vi "Cluster Typedef JSON Staging.vi"() -> ()   [LabVIEW 2016]
uses:
  <userlib>/LevyLab/Lockin-Multichannel/Typedefs/AO-cluster.ctl
  <userlib>/LevyLab/Lockin-Multichannel/Typedefs/AO_Amp-array.ctl
  <userlib>/LevyLab/Lockin-Multichannel/Typedefs/AO_DC-array.ctl
  <userlib>/LevyLab/Lockin-Multichannel/Typedefs/AO_f-array.ctl
  <userlib>/LevyLab/Lockin-Multichannel/Typedefs/AO_phi-array.ctl
  <userlib>/LevyLab/Lockin-Multichannel/Typedefs/Function-array.ctl
  <userlib>/LevyLab/Lockin-Multichannel/Typedefs/Function-enum.ctl
  <userlib>/LevyLab/Krohn Hite 7008/typedefs/KH_control_array.ctl
  <userlib>/LevyLab/Krohn Hite 7008/typedefs/KH_control.ctl
  <userlib>/LevyLab/Krohn Hite 7008/typedefs/Channel-Enum.ctl
  <userlib>/LevyLab/Krohn Hite 7008/typedefs/Gain-Enum.ctl
  <userlib>/LevyLab/Krohn Hite 7008/typedefs/Shunt-Enum.ctl
  <userlib>/LevyLab/Krohn Hite 7008/typedefs/Input Configuration-Enum.ctl
  <userlib>/LevyLab/Lockin-Multichannel/Typedefs/REF-cluster.ctl
  <userlib>/LevyLab/Lockin-Multichannel/Typedefs/REF_f-array.ctl
  <userlib>/LevyLab/Lockin-Multichannel/Typedefs/REF_phi-array.ctl
  <vilib>/addons/_JKI.lib/Serialization/JSON/JKI JSON Serialization.lvlib
  <userlib>/LevyLab/Krohn Hite 7008/KH7008.lvclass
panel:
  out "x = y?":T1
  out "from JSON (ms)":u32
  out "to JSON (ms)":u32
  out "JSON String":string
  in  "Experiment Description":T2
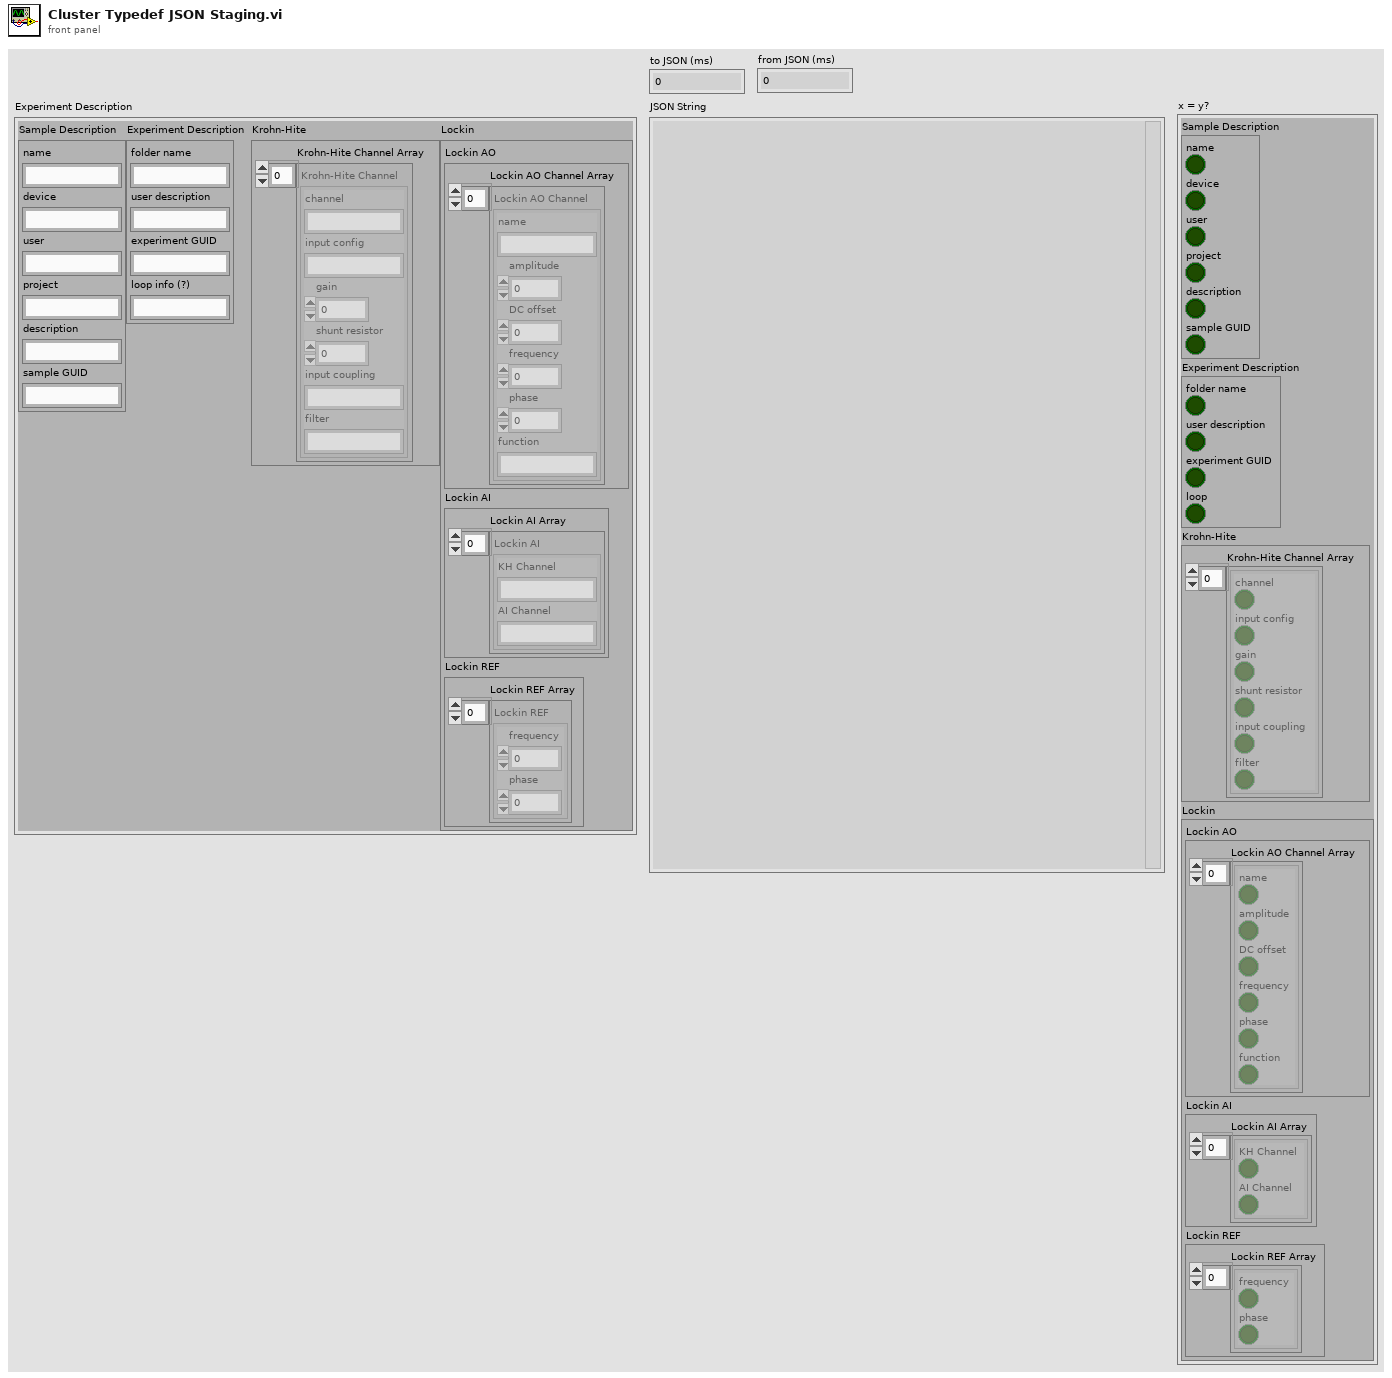
[diagram p1: front panel]
types:
  T1 = cluster{"Sample Description":cluster{"name":bool, "device":bool, "user":bool, "project":bool, "description":bool, "sample GUID":bool}, "Experiment Description":cluster{"folder name":bool, "user description":bool, "experiment GUID":bool, "loop":bool}, "Krohn-Hite":cluster{"Krohn-Hite Channel Array":cluster{"channel":bool, "input config":bool, "gain":bool, "shunt resistor":bool, "input coupling":bool, "filter":bool}[]}, "Lockin":cluster{"Lockin AO":cluster{"Lockin AO Channel Array":cluster{"name":bool, "amplitude":bool, "DC offset":bool, "frequency":bool, "phase":bool, "function":bool}[]}, "Lockin AI":cluster{"Lockin AI Array":cluster{"KH Channel":bool, "AI Channel":bool}[]}, "Lockin REF":cluster{"Lockin REF Array":cluster{"frequency":bool, "phase":bool}[]}}}
  T2 = cluster{"Sample Description":cluster{"name":string, "device":string, "user":string, "project":string, "description":string, "sample GUID":string}, "Experiment Description":cluster{"folder name":string, "user description":string, "experiment GUID":string, "loop info (?)":string}, "Krohn-Hite":cluster{"Krohn-Hite Channel Array":cluster{"channel":string, "input config":string, "gain":i32, "shunt resistor":i32, "input coupling":string, "filter":string}[]}, "Lockin":cluster{"Lockin AO":cluster{"Lockin AO Channel Array":cluster{"name":string, "amplitude":dbl, "DC offset":dbl, "frequency":dbl, "phase":dbl, "function":string}[]}, "Lockin AI":cluster{"Lockin AI Array":cluster{"KH Channel":string, "AI Channel":string}[]}, "Lockin REF":cluster{"Lockin REF Array":cluster{"frequency":dbl, "phase":dbl}[]}}}
  T3 = typedef "REF-cluster.ctl" = cluster{"REF f (Hz)":T4, "REF phi (°)":T5}
  T4 = typedef "REF_f-array.ctl" = dbl[]
  T5 = typedef "REF_phi-array.ctl" = dbl[]
  T6 = typedef "KH7008.lvclass/KH_control_array.ctl" = T7[]
  T7 = typedef "KH7008.lvclass/KH_control.ctl" = cluster{"Channel":T8, "Gain":T9, "Shunt Resistor":T10, "Input Config":T11}
  T8 = typedef "KH7008.lvclass/Channel-Enum.ctl" = enum16{"Channel 1", "Channel 2", "Channel 3", "Channel 4", "Channel 5", "Channel 6", "Channel 7", "Channel 8"}
  T9 = typedef "KH7008.lvclass/Gain-Enum.ctl" = enum16{"1x", "10x", "100x", "1000x"}
  T10 = typedef "KH7008.lvclass/Shunt-Enum.ctl" = enum16{"Open", "50 Ohms", "500 Ohms", "5k Ohms", "50k Ohms"}
  T11 = typedef "KH7008.lvclass/Input Configuration-Enum.ctl" = enum16{"Ground", "SE+ (-gnd)", "SE- (+gnd)", "Differential"}
  T12 = typedef "AO-cluster.ctl" = cluster{"AO amp (V)":T13, "AO DC (V)":T14, "AO f (Hz)":T15, "AO phi (°)":T16, "function":T17, "I+":bool[]}
  T13 = typedef "AO_Amp-array.ctl" = dbl[]
  T14 = typedef "AO_DC-array.ctl" = dbl[]
  T15 = typedef "AO_f-array.ctl" = dbl[]
  T16 = typedef "AO_phi-array.ctl" = dbl[]
  T17 = typedef "Function-array.ctl" = T18[]
  T18 = typedef "Function-enum.ctl" = enum16{"Sine", "Triangle", "Square", "Sawtooth"}
  T19 = cluster{"name":string, "device":string, "user":string, "project":string, "description":string, "sample GUID":string}
  T20 = cluster{"folder name":string, "user description":string, "experiment GUID":string, "loop info (?)":string}
  T21 = cluster{"Krohn-Hite Channel Array":cluster{"channel":string, "input config":string, "gain":i32, "shunt resistor":i32, "input coupling":string, "filter":string}[]}
  T22 = cluster{"Lockin AO":cluster{"Lockin AO Channel Array":cluster{"name":string, "amplitude":dbl, "DC offset":dbl, "frequency":dbl, "phase":dbl, "function":string}[]}, "Lockin AI":cluster{"Lockin AI Array":cluster{"KH Channel":string, "AI Channel":string}[]}, "Lockin REF":cluster{"Lockin REF Array":cluster{"frequency":dbl, "phase":dbl}[]}}
  T23 = cluster{"channel":string, "input config":string, "gain":i32, "shunt resistor":i32, "input coupling":string, "filter":string}[]
  T24 = cluster{"channel":string, "input config":string, "gain":i32, "shunt resistor":i32, "input coupling":string, "filter":string}
  T25 = cluster{"Lockin REF Array":cluster{"frequency":dbl, "phase":dbl}[]}
  T26 = cluster{"Lockin AI Array":cluster{"KH Channel":string, "AI Channel":string}[]}
  T27 = cluster{"KH Channel":string, "AI Channel":string}[]
  T28 = cluster{"KH Channel":string, "AI Channel":string}
  T29 = cluster{"Lockin AO Channel Array":cluster{"name":string, "amplitude":dbl, "DC offset":dbl, "frequency":dbl, "phase":dbl, "function":string}[]}
  T30 = cluster{"name":string, "amplitude":dbl, "DC offset":dbl, "frequency":dbl, "phase":dbl, "function":string}[]
  T31 = cluster{"name":string, "amplitude":dbl, "DC offset":dbl, "frequency":dbl, "phase":dbl, "function":string}
  T32 = cluster{"Sample Description":cluster{"name":bool, "device":bool, "user":bool, "project":bool, "description":bool, "sample GUID":bool}, "Experiment Description":cluster{"folder name":bool, "user description":bool, "experiment GUID":bool, "loop info (?)":bool}, "Krohn-Hite":cluster{"Krohn-Hite Channel Array":cluster{"channel":bool, "input config":bool, "gain":bool, "shunt resistor":bool, "input coupling":bool, "filter":bool}[]}, "Lockin":cluster{"Lockin AO":cluster{"Lockin AO Channel Array":cluster{"name":bool, "amplitude":bool, "DC offset":bool, "frequency":bool, "phase":bool, "function":bool}[]}, "Lockin AI":cluster{"Lockin AI Array":cluster{"KH Channel":bool, "AI Channel":bool}[]}, "Lockin REF":cluster{"Lockin REF Array":cluster{"frequency":bool, "phase":bool}[]}}}
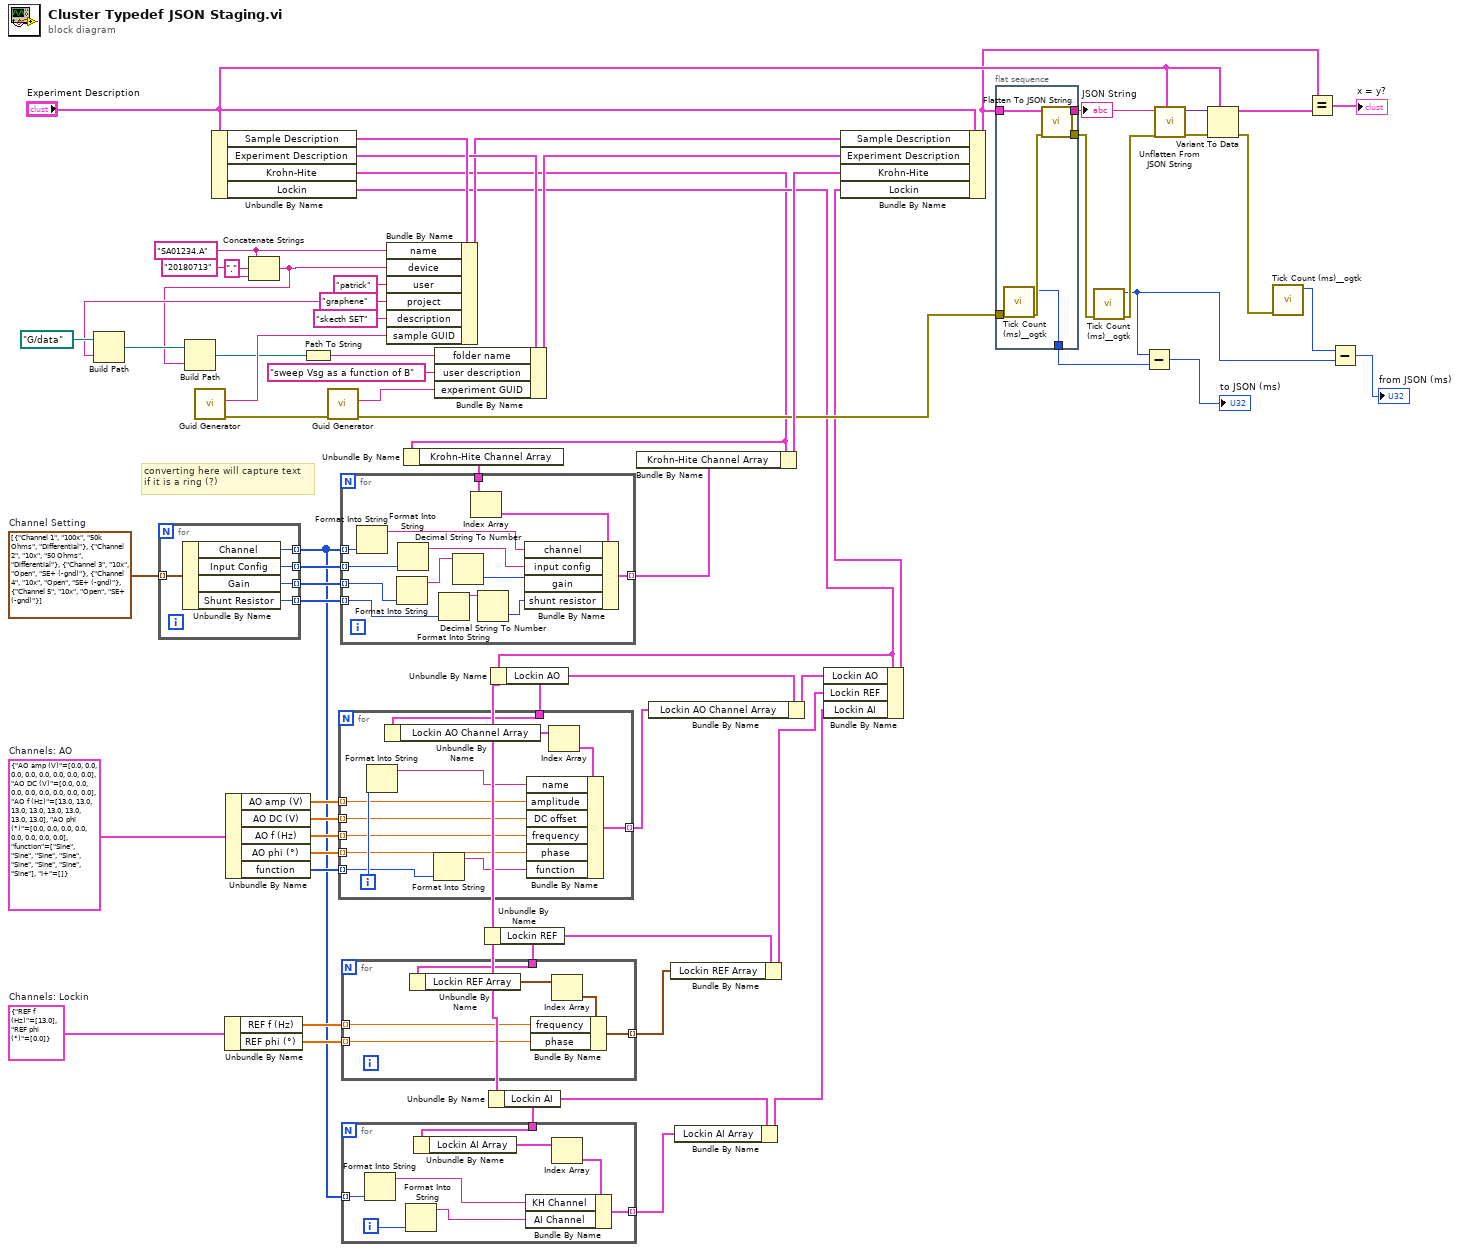
[diagram p0: block diagram]
diagram:
  w16 = T3 {"REF f (Hz)"=[13.0], "REF phi (°)"=[0.0]}  # Channels: Lockin
  w39 = "SA01234.A" ("name")
  w3 = "graphene" ("project")
  w60 = T6 [{"Channel"=enum."Channel 1", "Gain"=enum."100x", "Shunt Resistor"=enum."50k Ohms", "Input Config"=enum."Differential"}, {"Channel"=enum."Channel 2", "Gain"=enum."10x", "Shunt Resistor"=enum."50 Ohms", "Input Config"=enum."Differential"}, {"Channel"=enum."Channel 3", "Gain"=enum."10x", "Shunt Resistor"=enum."Open", "Input Config"=enum."SE+ (-gnd)"}, {"Channel"=enum."Channel 4", "Gain"=enum."10x", "Shunt Resistor"=enum."Open", "Input Config"=enum."SE+ (-gnd)"}, {"Channel"=enum."Channel 5", "Gain"=enum."10x", "Shunt Resistor"=enum."Open", "Input Config"=enum."SE+ (-gnd)"}]  # Channel Setting
  w53 = T12 {"AO amp (V)"=[0.0, 0.0, 0.0, 0.0, 0.0, 0.0, 0.0, 0.0], "AO DC (V)"=[0.0, 0.0, 0.0, 0.0, 0.0, 0.0, 0.0, 0.0], "AO f (Hz)"=[13.0, 13.0, 13.0, 13.0, 13.0, 13.0, 13.0, 13.0], "AO phi (°)"=[0.0, 0.0, 0.0, 0.0, 0.0, 0.0, 0.0, 0.0], "function"=[enum."Sine", enum."Sine", enum."Sine", enum."Sine", enum."Sine", enum."Sine", enum."Sine", enum."Sine"], "I+"=[]}  # Channels: AO
  # "converting here will capture text\nif it is a ring (?)"
  n1 = Build Path(base path=path "G:/data", name or relative path=w3) -> (appended path=w35:path)
  n2 = for {
    tunnel: w60 -> [w69] mode=indexing
    tunnel: [w68] -> w1 mode=indexing
    tunnel: [w67] -> w59 mode=indexing
    tunnel: [w66] -> w58 mode=indexing
    tunnel: [w65] -> w57 mode=indexing
    n3 = Unbundle By Name(w69) -> ("Channel"=w68:T8, "Input Config"=w67:T11, "Gain"=w66:T9, "Shunt Resistor"=w65:T10)
  }
  n4 = call <vilib>:"Guid Generator.vi"() -> ("error out"=w19:errorcluster, "GUID"=w37:string)  [unwired: 10 in]
  n5 = Unbundle By Name("Experiment Description") -> ("Sample Description"=w64:T19, "Experiment Description"=w62:T20, "Krohn-Hite"=w6:T21, "Lockin"=w8:T22)
  n6 = Unbundle By Name(w16) -> ("REF f (Hz)"=w15:T4, "REF phi (°)"=w14:T5)
  n7 = Unbundle By Name(w53) -> ("AO amp (V)"=w52:T13, "AO DC (V)"=w51:T14, "AO f (Hz)"=w48:T15, "AO phi (°)"=w47:T16, "function"=w46:T17)
  n8 = Concatenate Strings(w39, "." ("string"), "20180713" ("device")) -> (w2:string)
  n9 = Build Path(base path=w35, name or relative path=w2) -> (appended path=w34:path)
  n10 = Path To String(path=w34) -> (string=w33:string)
  n11 = call <vilib>:"Guid Generator.vi"("error in (no error)"=w19) -> ("error out"=w18:errorcluster, "GUID"=w45:string)  [unwired: 9 in]
  n12 = Bundle By Name(cluster=w64, "name"=w39, "device"=w2, "user"="patrick", "project"=w3, "description"="skecth SET", "sample GUID"=w37) -> (w56:T19)
  n13 = Unbundle By Name(w6) -> ("Krohn-Hite Channel Array"=w55:T23)
  n14 = for {
    tunnel: w55 -> [w79]
    tunnel: [w82] -> w54 mode=indexing
    tunnel: w1 -> [w81] mode=indexing
    tunnel: w59 -> [w80] mode=indexing
    tunnel: w58 -> [w75] mode=indexing
    tunnel: w57 -> [w74] mode=indexing
    n15 = Format Into String(w81) -> (resulting string=w76:string)  [unwired: 3 in, 1 out]
    n16 = Format Into String(w75) -> (resulting string=w72:string)  [unwired: 3 in, 1 out]
    n17 = Format Into String(w80) -> (resulting string=w77:string)  [unwired: 3 in, 1 out]
    n18 = Format Into String(w74) -> (resulting string=w73:string)  [unwired: 3 in, 1 out]
    n19 = Decimal String To Number(string=w72) -> (number=w71:i32)  [unwired: 2 in, 1 out]
    n20 = Index Array(array=w79) -> (element=w78:T24)  [unwired: 1 in]
    n21 = Decimal String To Number(string=w73) -> (number=w70:i32)  [unwired: 2 in, 1 out]
    n22 = Bundle By Name(cluster=w78, "channel"=w76, "input config"=w77, "gain"=w71, "shunt resistor"=w70) -> (w82:T24)
  }
  n23 = Bundle By Name(cluster=w62, "folder name"=w33, "user description"="sweep Vsg as a function of B" ("description"), "experiment GUID"=w45) -> (w63:T20)
  n24 = Unbundle By Name(w8) -> ("Lockin REF"=w13:T25)
  n25 = for {
    tunnel: w13 -> [w87]
    tunnel: [w88] -> w12 mode=indexing
    tunnel: w15 -> [w84] mode=indexing
    tunnel: w14 -> [w83] mode=indexing
    n26 = Unbundle By Name(w87) -> ("Lockin REF Array"=w86:cluster{"frequency":dbl, "phase":dbl}[])
    n27 = Index Array(array=w86) -> (element=w85:cluster{"frequency":dbl, "phase":dbl})  [unwired: 1 in]
    n28 = Bundle By Name(cluster=w85, "frequency"=w84, "phase"=w83) -> (w88:cluster{"frequency":dbl, "phase":dbl})
  }
  n29 = Unbundle By Name(w8) -> ("Lockin AI"=w9:T26)
  n30 = for {
    tunnel: w9 -> [w95]
    tunnel: [w96] -> w10 mode=indexing
    tunnel: w1 -> [w91] mode=indexing
    i -> [w92]
    n31 = Format Into String(w91) -> (resulting string=w89:string)  [unwired: 3 in, 1 out]
    n32 = Format Into String(w92) -> (resulting string=w90:string)  [unwired: 3 in, 1 out]
    n33 = Unbundle By Name(w95) -> ("Lockin AI Array"=w94:T27)
    n34 = Index Array(array=w94) -> (element=w93:T28)  [unwired: 1 in]
    n35 = Bundle By Name(cluster=w93, "KH Channel"=w89, "AI Channel"=w90) -> (w96:T28)
  }
  n36 = Unbundle By Name(w8) -> ("Lockin AO"=w50:T29)
  n37 = for {
    tunnel: w50 -> [w103]
    tunnel: [w108] -> w4 mode=indexing
    tunnel: w52 -> [w105] mode=indexing
    tunnel: w51 -> [w104] mode=indexing
    tunnel: w48 -> [w100] mode=indexing
    tunnel: w47 -> [w99] mode=indexing
    tunnel: w46 -> [w98] mode=indexing
    i -> [w106]
    n38 = Format Into String(w106) -> (resulting string=w107:string)  [unwired: 3 in, 1 out]
    n39 = Unbundle By Name(w103) -> ("Lockin AO Channel Array"=w102:T30)
    n40 = Format Into String(w98) -> (resulting string=w97:string)  [unwired: 3 in, 1 out]
    n41 = Index Array(array=w102) -> (element=w101:T31)  [unwired: 1 in]
    n42 = Bundle By Name(cluster=w101, "name"=w107, "amplitude"=w105, "DC offset"=w104, "frequency"=w100, "phase"=w99, "function"=w97) -> (w108:T31)
  }
  n43 = Bundle By Name(cluster=w6, "Krohn-Hite Channel Array"=w54) -> (w61:T21)
  n44 = Bundle By Name(cluster=w50, "Lockin AO Channel Array"=w4) -> (w49:T29)
  n45 = Bundle By Name(cluster=w13, "Lockin REF Array"=w12) -> (w11:T25)
  n46 = Bundle By Name(cluster=w9, "Lockin AI Array"=w10) -> (w7:T26)
  n47 = Bundle By Name(cluster=w8, "Lockin AO"=w49, "Lockin REF"=w11, "Lockin AI"=w7) -> (w17:T22)
  n48 = Bundle By Name(cluster="Experiment Description", "Sample Description"=w56, "Experiment Description"=w63, "Krohn-Hite"=w61, "Lockin"=w17) -> (w23:T2)
  n49 = flat-sequence {
    tunnel: [w114] -> w36
    tunnel: [w112] -> w29
    tunnel: w23 -> [w111]
    tunnel: [w110] -> w22
    tunnel: w18 -> [w109]
    frame #0 {
      n50 = call <userlib>:"Tick Count (ms)__ogtk.vi"("error in (no error)"=w109) -> ("error out"=w113:errorcluster, "millisecond timer value"=w110:u32)  [unwired: 9 in]
      n51 = call <vilib>:"Flatten To JSON String.vi"("error in (no error)"=w113, "Variant"=w111) -> ("error out"=w112:errorcluster, "JSON String"=w114:string)  [unwired: 8 in]
    }
  }
  n52 = call <userlib>:"Tick Count (ms)__ogtk.vi"("error in (no error)"=w29) -> ("error out"=w28:errorcluster, "millisecond timer value"=w20:u32)  [unwired: 9 in]
  n53 = Subtract(x=w20, y=w22) -> (x-y=→"to JSON (ms)":u32)
  n54 = call <vilib>:"Unflatten From JSON String.vi"("Type and Defaults"="Experiment Description", "error in (no error)"=w28, "JSON String"=w36) -> ("error out"=w32:errorcluster, "Variant"=w31:variant)  [unwired: 7 in]
  n55 = Variant To Data(error in=w32, type="Experiment Description", Variant=w31) -> (data=w24:T2, error out=w27:errorcluster)
  n56 = call <userlib>:"Tick Count (ms)__ogtk.vi"("error in (no error)"=w27) -> ("millisecond timer value"=w21:u32)  [unwired: 9 in, 1 out]
  n57 = Equal?(x=w23, y=w24) -> (x = y?=→"x = y?":T32)
  n58 = Subtract(x=w21, y=w20) -> (x-y=→"from JSON (ms)":u32)
  "JSON String" <- w36
